vi "Get Pin Status Response.vi"(8 "error in (no error)":errorcluster, 11 "NXP in":refnum<class "NXP.lvclass">) -> (0 "error out":errorcluster, 2 "Value":string, 3 "NXP out":refnum<class "NXP.lvclass">)   [LabVIEW 2020, in "NXP.lvclass"]
uses:
  NXP.lvclass
  Abstract/Serial device/Serial device.lvclass
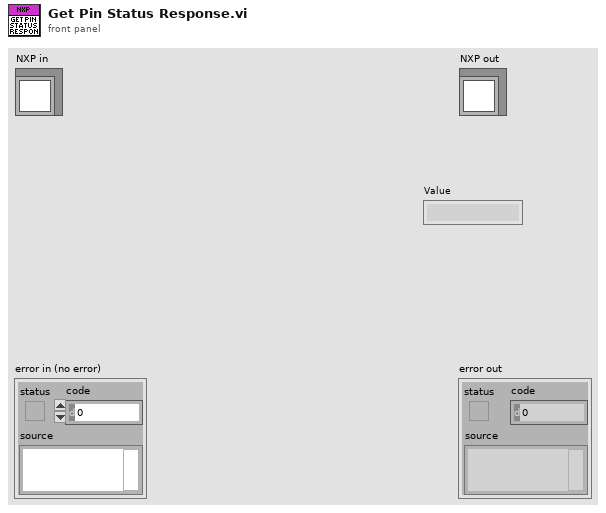
[diagram p1: front panel]
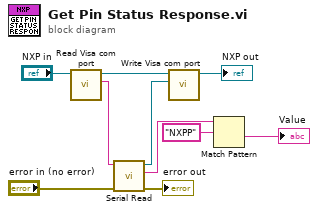
[diagram p0: block diagram]
diagram:
  n1 = call-dynamic "Read Visa com port.vi"("Serial device in"="NXP in") -> ("Visa com port"=w10:string, "Serial device out"=w8:refnum<class "NXP.lvclass">)  [unwired: 8 in, 1 out]
  n2 = call "Serial Read.vi"("error in (no error)"="error in (no error)", "VISA resource name in"=w10) -> ("error out"=→"error out":errorcluster, "Serial Response"=w3:string, "VISA resource name out"=w9:refnum<visa-resource-name>)  [unwired: 7 in]
  n3 = call-dynamic "Write Visa com port.vi"("Visa com port"=w9, "Serial device in"=w8) -> ("Serial device out"=→"NXP out":refnum<class "NXP.lvclass">)  [unwired: 8 in, 1 out]
  n4 = Match Pattern(string=w3, regular expression="NXPP") -> (after substring=→"Value":string)  [unwired: 1 in, 3 out]
